vi "Send Async ACQ Notification.vi"(8 "error in (no error)":errorcluster, 10 "Async ACQ":T1, 11 "Async ACQ Notifier in":refnum<notifier>) -> (0 "error out":errorcluster, 3 "Async ACQ Notifier out":refnum<notifier>)   [LabVIEW 2014, in "WINFAS 2 Data Queue.lvlib"]
uses:
  WINFAS 2 Data Queue.lvlib
  Async Acquisition Data Cluster.ctl
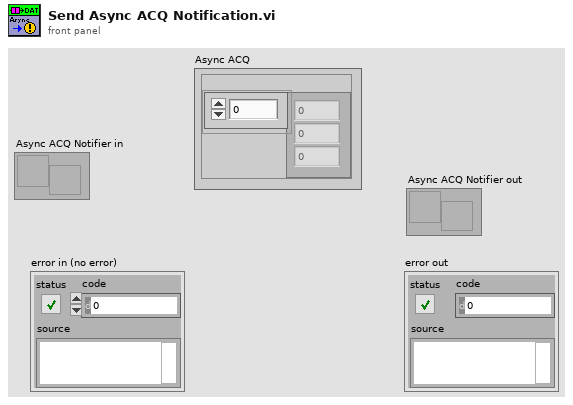
[diagram p1: front panel]
types:
  T1 = typedef "WINFAS 2 Data Queue.lvlib/Async Acquisition Data Cluster.ctl" = cluster{"Data":sgl[]}
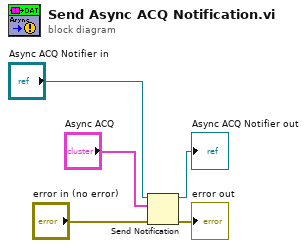
[diagram p0: block diagram]
diagram:
  n1 = Send Notification(notification="Async ACQ", notifier="Async ACQ Notifier in", error in (no error)="error in (no error)") -> (notifier out=→"Async ACQ Notifier out":refnum<notifier>, error out=→"error out":errorcluster)
